vi "RemoveByName.vi"(10 "Nominal Points in":T2(array[cluster]), 11 "Nominal to be Removes":string) -> (3 "Nominal Points out":T2(array[cluster]))   [LabVIEW 2017]
uses:
  AT901 API/Structures/Struct TransformationPoint.ctl
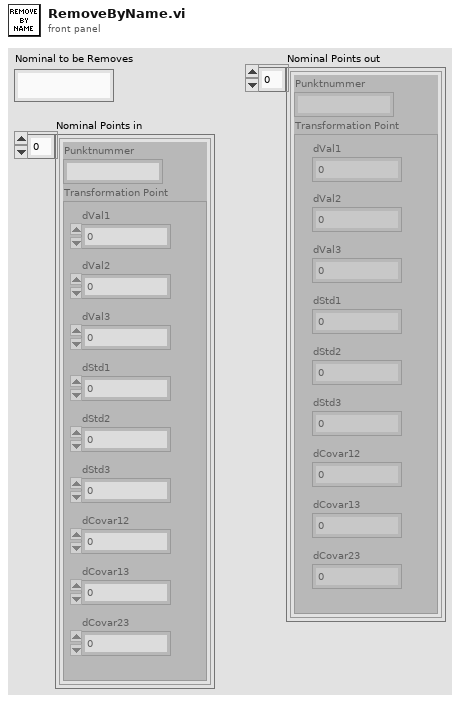
[diagram p1: front panel]
types:
  T1 = typedef "Struct TransformationPoint.ctl" = cluster{"dVal1":dbl, "dVal2":dbl, "dVal3":dbl, "dStd1":dbl, "dStd2":dbl, "dStd3":dbl, "dCovar12":dbl, "dCovar13":dbl, "dCovar23":dbl}
  T2 = cluster{"Punktnummer":string, "Transformation Point":T1}[]
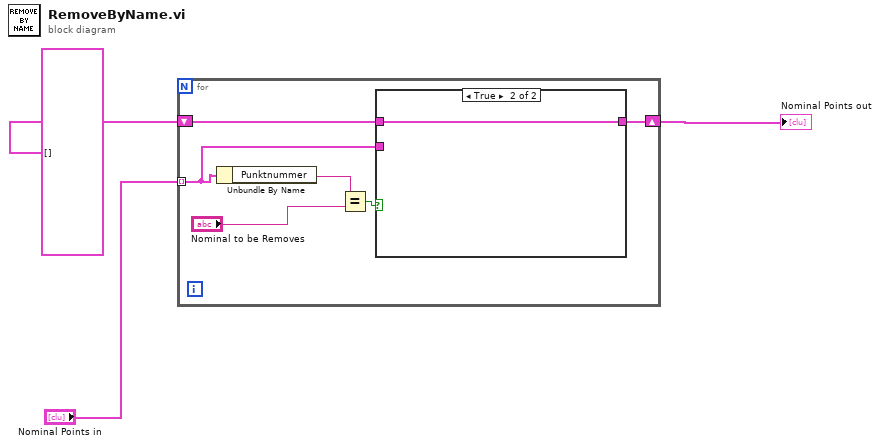
[diagram p0: block diagram]
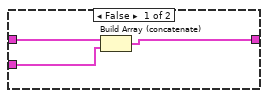
[diagram p2: hidden frame]
diagram:
  n1 = for {
    tunnel: "Nominal Points in" -> [w5] mode=indexing
    shift-right: [w4] -> w3
    shift-left: T2 [] ("Nominal Points") -> [w6]
    n2 = Unbundle By Name(w5) -> ("Punktnummer"=w9:string)
    n3 = Equal?(x=w9, y="Nominal to be Removes") -> (x = y?=w7:bool)
    n4 = case shown="True" w7 {
      tunnel: w6 -> [w11 w13]
      tunnel: [w10 w13] -> w4
      tunnel: w5 -> [w12 _]
      frame False {
        n5 = Build Array (concatenate)(w11, w12) -> (w10:T2)
      }
      frame True {
      }
    }
  }
  "Nominal Points out" <- w3
